vi "Data_GetStreamInfo.vi"(8 "error in (no error)":errorcluster, 11 "data":variant) -> (0 "error out":errorcluster, 1 "block":i32, 2 "stream Id":string, 3 "found":bool)   [LabVIEW 2017, in "FileManager.lvlib"]
uses:
  <vilib>/addons/InsightCM/Devices/Shared/Common/FileManager/FileManager.lvlib
  <vilib>/addons/InsightCM/Devices/Shared/Common/FileManager/controls/DataPropertyNames.ctl
panel:
  out "data out":variant
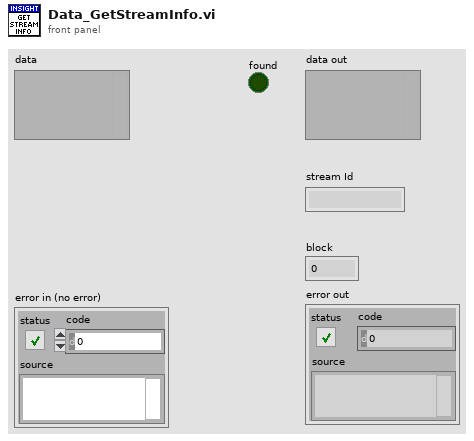
[diagram p1: front panel]
types:
  T1 = typedef "DataPropertyNames.ctl" = enum16{"Type", "EventRef", "FilePath", "DataGroup", "AcquisitionTimestamp", "StreamId", "StreamBlock", "TrendPointsOnly", "ExtraLargeFile"}
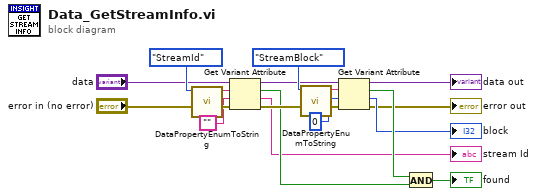
[diagram p0: block diagram]
diagram:
  n1 = call <vilib>:"DataPropertyEnumToString.vi"("property"=DataPropertyNames."StreamId" ("Names")) -> ("string"=w13:string)  [unwired: 10 in]
  n2 = Get Variant Attribute(Variant="data", name=w13, default value (empty Variant)="", error in="error in (no error)") -> (duplicate Variant=w12:variant, found=w7:bool, value=→"stream Id":string, error out=w9:errorcluster)
  n3 = call <vilib>:"DataPropertyEnumToString.vi"("property"=DataPropertyNames."StreamBlock" ("Names")) -> ("string"=w11:string)  [unwired: 10 in]
  n4 = Get Variant Attribute(Variant=w12, name=w11, default value (empty Variant)=0, error in=w9) -> (duplicate Variant=→"data out":variant, found=w8:bool, value=→"block":i32, error out=→"error out":errorcluster)
  n5 = And(x=w8, y=w7) -> (x .and. y?=→"found":bool)
